vi "createInterface.vi"() -> ()   [LabVIEW 2018, in "MotorControllerClass.lvclass"]
uses:
  BMS/MotorControllerClass.lvclass
  <vilib>/CANopenLib/CANOPEN.llb/CANopen Interface Create.vi
panel:
  in  "MotorControllerClass in":refnum<class "MotorControllerClass.lvclass">
  out "MotorControllerClass out":refnum<class "MotorControllerClass.lvclass">
  out "interface object out":refnum<k20>
  out "error out":errorcluster
  in  "error in (no error)":errorcluster
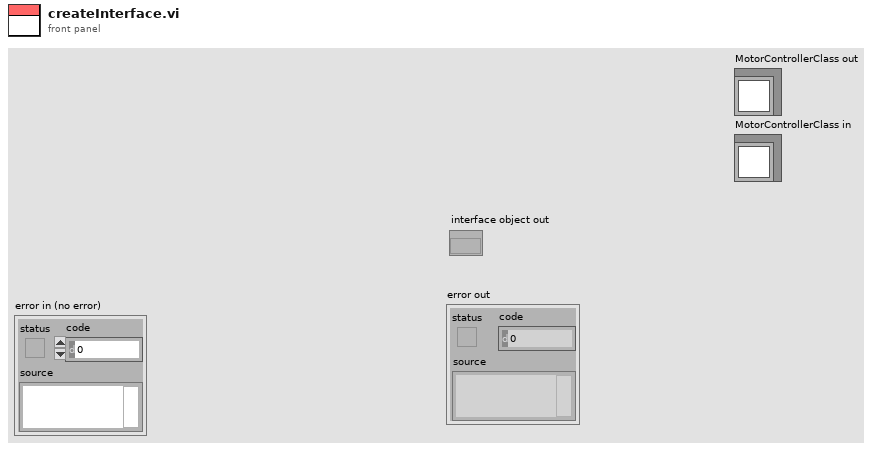
[diagram p1: front panel]
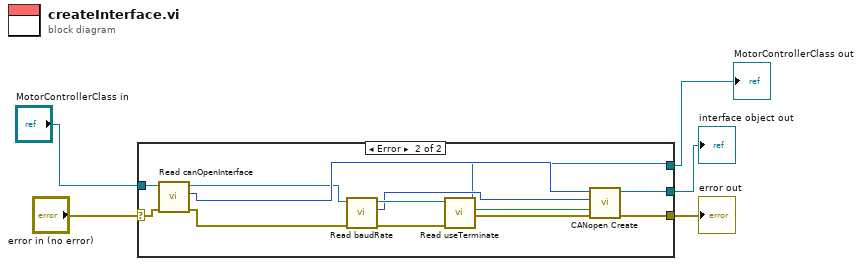
[diagram p0: block diagram]
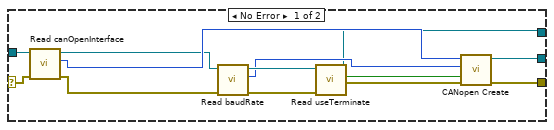
[diagram p2: hidden frame]
diagram:
  n1 = case shown="Error" "error in (no error)" {
    selector: "error in (no error)" -> [w15 w28]
    tunnel: [w17 w30] -> w4
    tunnel: [w18 w31] -> w3
    tunnel: [w7 w20] -> w1
    tunnel: "MotorControllerClass in" -> [w6 w19]
    frame No Error {
      n2 = call-dynamic "Read canOpenInterface.vi"("error in (no error)"=w15, "MotorControllerClass in"=w6) -> ("error out"=w13:errorcluster, "canOpenInterface"=w16:u32, "MotorControllerClass out"=w14:refnum<class "MotorControllerClass.lvclass">)  [unwired: 7 in]
      n3 = call-dynamic "Read baudRate.vi"("error in (no error)"=w13, "MotorControllerClass in"=w14) -> ("error out"=w12:errorcluster, "baudRate"=w8:u32, "MotorControllerClass out"=w11:refnum<class "MotorControllerClass.lvclass">)  [unwired: 7 in]
      n4 = call-dynamic "Read useTerminate.vi"("error in (no error)"=w12, "MotorControllerClass in"=w11) -> ("error out"=w10:errorcluster, "useTerminate"=w9:bool, "MotorControllerClass out"=w7:refnum<class "MotorControllerClass.lvclass">)  [unwired: 7 in]
      n5 = call-poly <vilib>:"CANopen Create.vi"("error in (no error)"=w10, "termination? (F)"=w9, "baud rate"=w8, "interface name"=w16) -> ("error out"=w17:errorcluster, "interface object out"=w18:refnum<k20>)  [unwired: 6 in]
    }
    frame Error {
      n6 = call-dynamic "Read canOpenInterface.vi"("error in (no error)"=w28, "MotorControllerClass in"=w19) -> ("error out"=w26:errorcluster, "canOpenInterface"=w29:u32, "MotorControllerClass out"=w27:refnum<class "MotorControllerClass.lvclass">)  [unwired: 7 in]
      n7 = call-dynamic "Read baudRate.vi"("error in (no error)"=w26, "MotorControllerClass in"=w27) -> ("error out"=w25:errorcluster, "baudRate"=w21:u32, "MotorControllerClass out"=w24:refnum<class "MotorControllerClass.lvclass">)  [unwired: 7 in]
      n8 = call-dynamic "Read useTerminate.vi"("error in (no error)"=w25, "MotorControllerClass in"=w24) -> ("error out"=w23:errorcluster, "useTerminate"=w22:bool, "MotorControllerClass out"=w20:refnum<class "MotorControllerClass.lvclass">)  [unwired: 7 in]
      n9 = call-poly <vilib>:"CANopen Create.vi"("error in (no error)"=w23, "termination? (F)"=w22, "baud rate"=w21, "interface name"=w29) -> ("error out"=w30:errorcluster, "interface object out"=w31:refnum<k20>)  [unwired: 6 in]
    }
  }
  "error out" <- w4
  "interface object out" <- w3
  "MotorControllerClass out" <- w1
